vi "I2C EEPROM Write-and-Read.vi"() -> ()   [LabVIEW 2020]
panel:
  in  "Read EEPROM":bool=TRUE
  in  "Write EEPROM":bool=TRUE
  out "Registers Read":string[](array[string])
  out "Registers Written":string[](array[string])
  out "Results for Read":dbl[][](array[numeric]) format="%.2f"
  out "Results for Write":dbl[][](array[numeric]) format="%.2f"
  out "Error String":string
  out "ConnectionType Out":i32
  out "DeviceType Out":i32
  in  "Identifier":string="LJM_idANY"
  in  "ConnectionType":string="LJM_ctANY"
  in  "DeviceType":string="LJM_dtANY"
  out "error out":errorcluster
  # "Before running this program:\n1. Attach a LJTick-DAC to FIO0 and FIO1\n\nProgram reads and writes 2 bytes of data \nto/from the user accessable memory \n(Word Address 0) on the LJTick-DAC.  \nUses the EEPROM \"BYTE  WRITE\" \nand \"RANDOM READ\" Features.\n\nEEPROM is available at Slave Address 0x50 \nor d80."
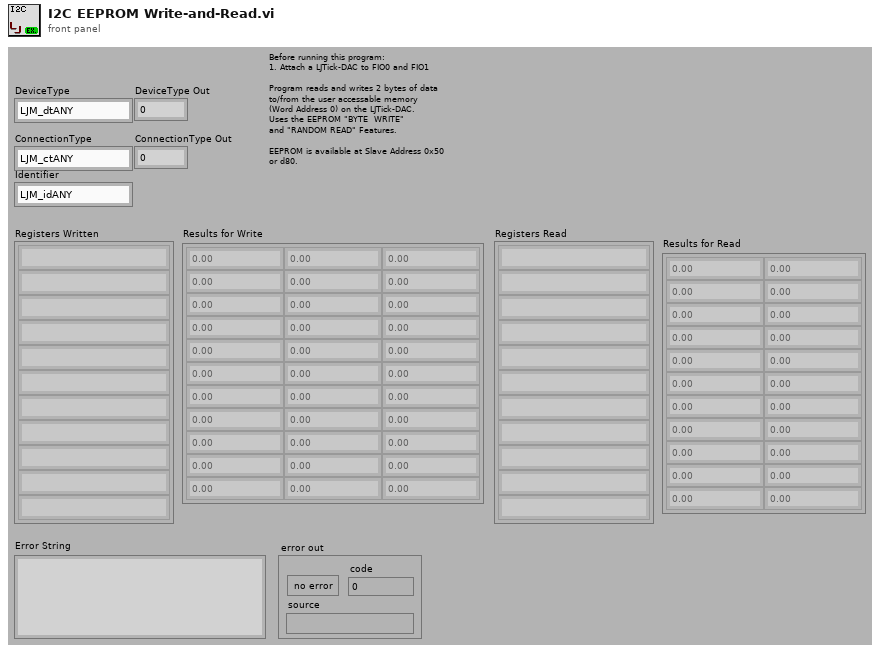
[diagram p1: front panel]
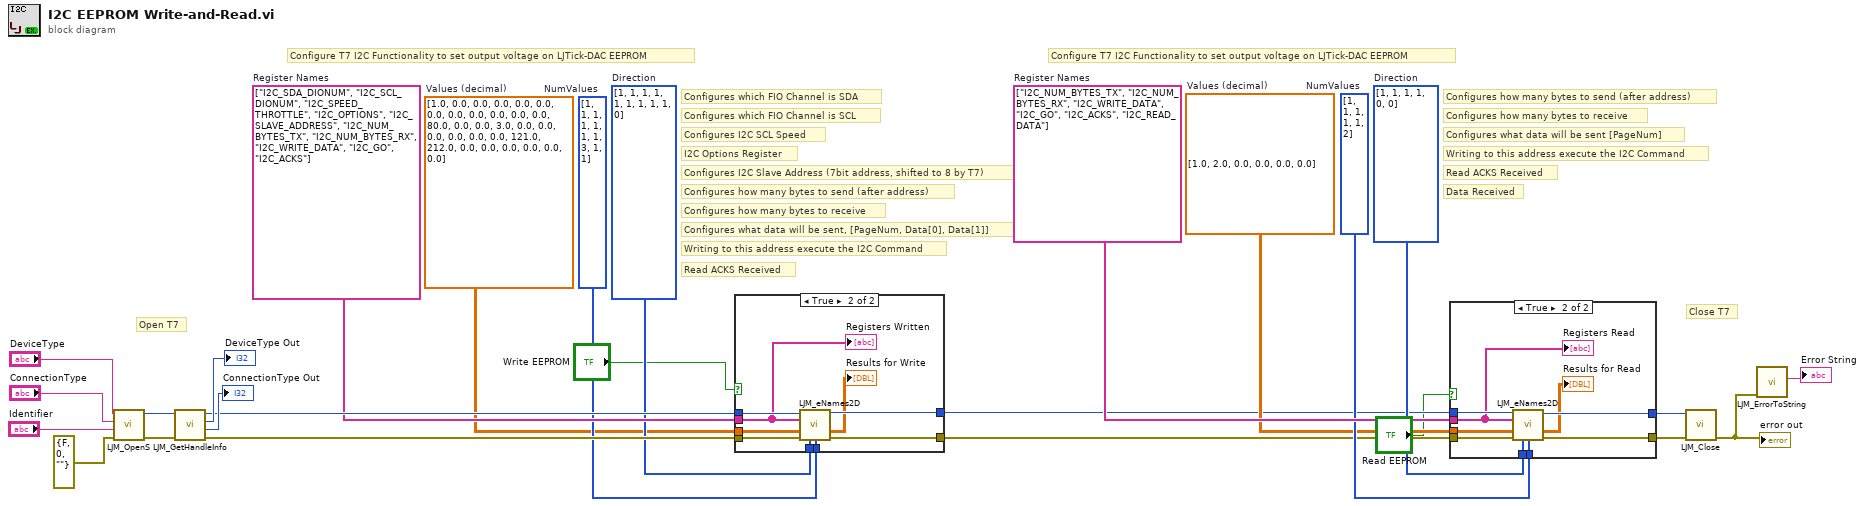
[diagram p0: block diagram]
diagram:
  w7 = dbl[][] [[1.0], [2.0], [0.0], [0.0], [0.0], [0.0]]  # Values (decimal)
  w8 = i32[] [1, 1, 1, 1, 0, 0] items=["Read", "Write"]  # Direction
  w9 = i32[] [1, 1, 1, 1, 1, 2]  # NumValues
  w10 = string[] ["I2C_NUM_BYTES_TX", "I2C_NUM_BYTES_RX", "I2C_WRITE_DATA", "I2C_GO", "I2C_ACKS", "I2C_READ_DATA"]  # Register Names
  w11 = dbl[][] [[1.0, 0.0, 0.0], [0.0, 0.0, 0.0], [0.0, 0.0, 0.0], [0.0, 0.0, 0.0], [80.0, 0.0, 0.0], [3.0, 0.0, 0.0], [0.0, 0.0, 0.0], [0.0, 121.0, 212.0], [0.0, 0.0, 0.0], [0.0, 0.0, 0.0]]  # Values (decimal)
  w12 = i32[] [1, 1, 1, 1, 1, 1, 1, 1, 1, 0] items=["Read", "Write"]  # Direction
  w13 = i32[] [1, 1, 1, 1, 1, 1, 1, 3, 1, 1]  # NumValues
  w14 = string[] ["I2C_SDA_DIONUM", "I2C_SCL_DIONUM", "I2C_SPEED_THROTTLE", "I2C_OPTIONS", "I2C_SLAVE_ADDRESS", "I2C_NUM_BYTES_TX", "I2C_NUM_BYTES_RX", "I2C_WRITE_DATA", "I2C_GO", "I2C_ACKS"]  # Register Names
  # "Close T7"
  # "Data Received"
  # "Read ACKS Received"
  # "Read ACKS Received"
  # "Configures how many bytes to send (after address)"
  # "Configures how many bytes to receive"
  # "Configures what data will be sent [PageNum]"
  # "Writing to this address execute the I2C Command"
  # "Configure T7 I2C Functionality to set output voltage on LJTick-DAC EEPROM"
  # "Configures which FIO Channel is SDA"
  # "Configures which FIO Channel is SCL"
  # "Configures I2C SCL Speed"
  # "I2C Options Register"
  # "Configures I2C Slave Address (7bit address, shifted to 8 by T7)"
  # "Configures how many bytes to send (after address)"
  # "Configures how many bytes to receive"
  # "Configures what data will be sent, [PageNum, Data[0], Data[1]]"
  # "Writing to this address execute the I2C Command"
  # "Open T7"
  # "Configure T7 I2C Functionality to set output voltage on LJTick-DAC EEPROM"
  n1 = call "LJM_OpenS.vi"("error in"=errorcluster {"status"=FALSE, "code"=0, "source"=""} ("error in (no error)"), "Identifier"="Identifier", "ConnectionType"="ConnectionType", "DeviceType"="DeviceType") -> ("error out"=w25:errorcluster, "Handle"=w24:i32)  [unwired: 6 in]
  n2 = call "LJM_GetHandleInfo.vi"("error in"=w25, "Handle In"=w24) -> ("error out"=w16:errorcluster, "ConnectionType"=→"ConnectionType Out":i32, "DeviceType"=→"DeviceType Out":i32, "Handle Out"=w15:i32)  [unwired: 2 in, 4 out]
  n3 = case shown="True" "Write EEPROM" {
    tunnel: w16 -> [w27 w37]
    tunnel: w15 -> [w28 w36]
    tunnel: w14 -> [_ w29]
    tunnel: w13 -> [_ w35]
    tunnel: w12 -> [_ w34]
    tunnel: w11 -> [_ w33]
    tunnel: [w28 w32] -> w6
    tunnel: [w27 w31] -> w5
    frame False {
    }
    frame True {
      n4 = call "LJM_eNames2D.vi"("Handle In"=w36, "aNames"=w29, "aValuesIn"=w33, "error in"=w37, "aWrites"=w34, "aNumValues"=w35) -> ("Handle Out"=w32:i32, "aValuesOut"=→"Results for Write":dbl[][], "error out"=w31:errorcluster)  [unwired: 6 in, 1 out]
      "Registers Written" <- w29
    }
  }
  n5 = case shown="True" "Read EEPROM" {
    tunnel: w10 -> [_ w41]
    tunnel: w9 -> [_ w48]
    tunnel: w8 -> [_ w40]
    tunnel: w7 -> [_ w47]
    tunnel: w6 -> [w39 w46]
    tunnel: w5 -> [w38 w45]
    tunnel: [w39 w44] -> w4
    tunnel: [w38 w43] -> w3
    frame False {
    }
    frame True {
      n6 = call "LJM_eNames2D.vi"("Handle In"=w46, "aNames"=w41, "aValuesIn"=w47, "error in"=w45, "aWrites"=w40, "aNumValues"=w48) -> ("Handle Out"=w44:i32, "aValuesOut"=→"Results for Read":dbl[][], "error out"=w43:errorcluster)  [unwired: 6 in, 1 out]
      "Registers Read" <- w41
    }
  }
  n7 = call "LJM_Close.vi"("error in"=w3, "Handle"=w4) -> ("error out"=w18:errorcluster)  [unwired: 9 in]
  "error out" <- w18
  n8 = call "LJM_ErrorToString.vi"("error in"=w18) -> ("String"=→"Error String":string)  [unwired: 10 in]
